vi "Source Autorange.vi"(6 "Autorange (On)":bool=TRUE, 7 "Function (Current)":enum32{"Current", "Voltage"}(ring), 8 "error in (no error)":errorcluster, 9 "Channel (Channel A)":T1, 10 "Node In":string, 11 "VISA resource name":refnum<visa-resource-name>) -> (0 "error out":errorcluster, 2 "Node Out":string, 3 "VISA resource name out":refnum<visa-resource-name>, 4 "Command String":string)   [LabVIEW 2012, in "Keithley 2600 Series.lvlib"]
doc: "This VI turns the SMU's source autoranging on or off.\n\n<b>Functions and Attributes Used</b>\nsmuX.source.autorangeY"
uses:
  Keithley 2600 Series.lvlib
  Private/GlobalVariables.vi
  Channel.ctl
panel:
  # "(c) 2008 Keithley Instruments, Inc.  ALL RIGHTS RESERVED."
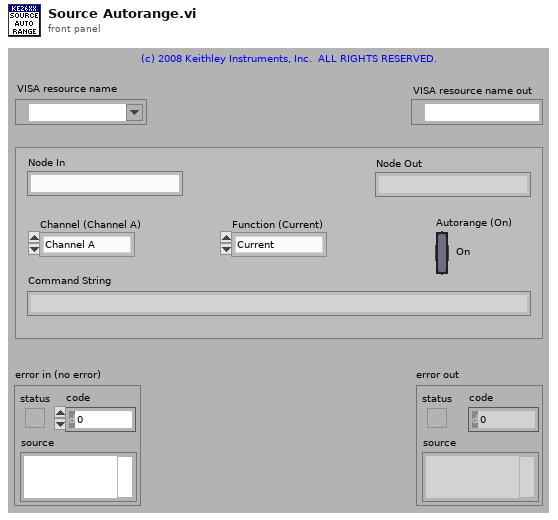
[diagram p1: front panel]
types:
  T1 = typedef "Keithley 2600 Series.lvlib/Channel.ctl" = enum32{"Channel A", "Channel B"}
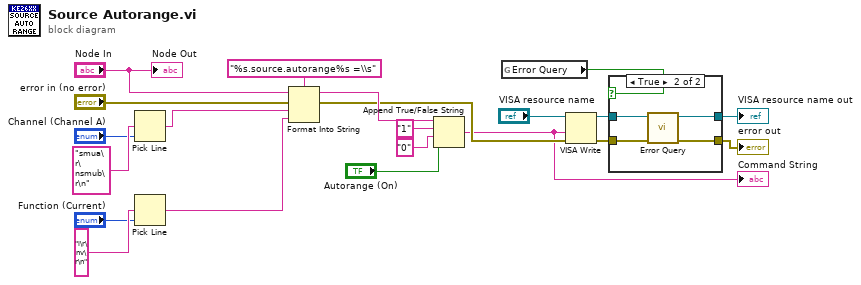
[diagram p0: block diagram]
diagram:
  n1 = Pick Line(multi-line string="smua\r\nsmub\r\n" ("options"), line index="Channel (Channel A)") -> (output string=w7:string)  [unwired: 1 out]
  n2 = Pick Line(multi-line string="i\r\nv\r\n" ("options"), line index="Function (Current)") -> (output string=w6:string)  [unwired: 1 out]
  n3 = Format Into String(format string="%s.source.autorange%s =\\s", initial string="Node In", error in="error in (no error)", w7, w6) -> (resulting string=w5:string, error out=w4:errorcluster)
  n4 = Append True/False String(1:"Autorange (On)", 2:"0" ("false string"), 3:"1" ("true string"), 4:w5) -> (0:w1:string)
  "Command String" <- w1
  n5 = global read "GlobalVariables.vi" "Error Query"() -> (w14:bool)
  n6 = VISA Write(VISA resource name="VISA resource name", write buffer=w1, error in (no error)=w4) -> (VISA resource name out=w13:refnum<visa-resource-name>, error out=w12:errorcluster)  [unwired: 1 out]
  n7 = case shown="True" w14 {
    tunnel: w13 -> [w23 w27]
    tunnel: w12 -> [w22 w26]
    tunnel: [w23 w25] -> w11
    tunnel: [w22 w24] -> w10
    frame False {
    }
    frame True {
      n8 = call "Error Query.vi"("error in (no error)"=w26, "VISA resource name"=w27) -> ("error out"=w24:errorcluster, "VISA resource name out"=w25:refnum<visa-resource-name>)  [unwired: 8 out]
    }
  }
  "VISA resource name out" <- w11
  "error out" <- w10
  "Node Out" <- "Node In"
